vi "AdjustWaveFormsLength.vi"(4 "error in (no error)":errorcluster, 7 "AllWaveFormsIN":waveform(dbl)[](graph)) -> (0 "error out":errorcluster, 3 "AllWaveFormsOUT":waveform(dbl)[](graph))   [LabVIEW 2017]
uses:
  <vilib>/Waveform/WDTOps.llb/WDT Waveform Duration DBL.vi
  <vilib>/Waveform/WDTOps.llb/WDT Get Waveform Subset DBL.vi
  <vilib>/Waveform/WDTOps.llb/WDT Align Waveform Timestamps DBL.vi
panel:
  out "waveforms out":waveform(dbl)[](array[waveform])
  out "ShortestDuration":dbl
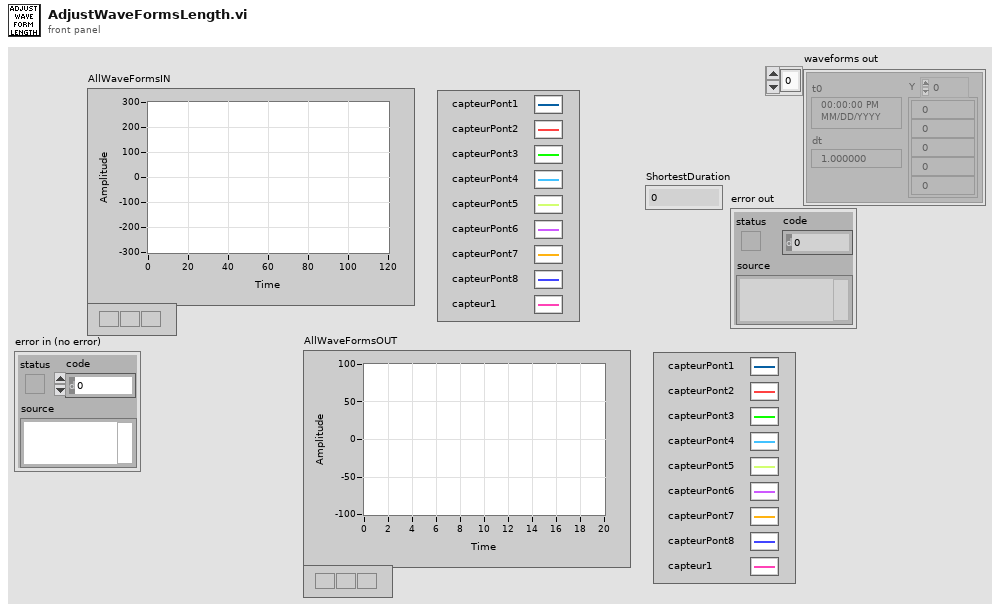
[diagram p1: front panel]
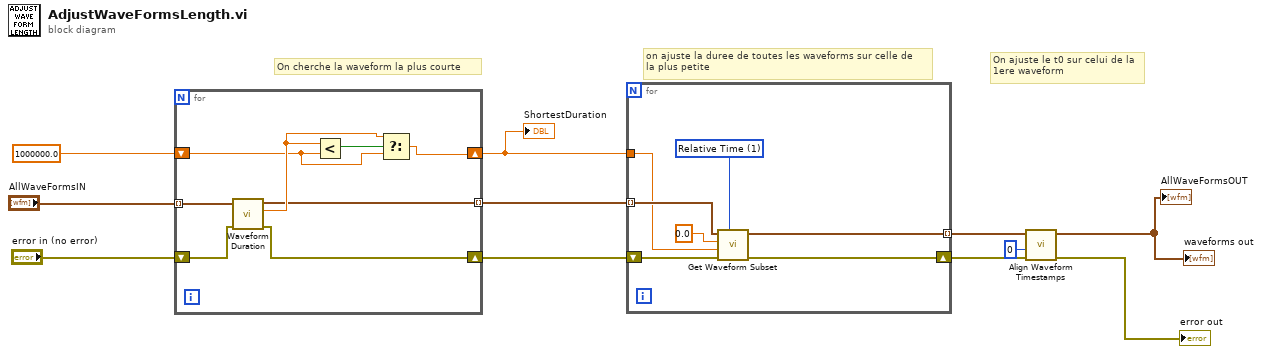
[diagram p0: block diagram]
diagram:
  # "On ajuste le t0 sur celui de la\n1ere waveform"
  # "on ajuste la duree de toutes les waveforms sur celle de\nla plus petite"
  # "On cherche la waveform la plus courte"
  n1 = for {
    tunnel: "AllWaveFormsIN" -> [w19] mode=indexing
    shift-right: [w17] -> w8
    shift-left: "error in (no error)" -> [w18]
    shift-right: [w14] -> w6
    shift-left: 1000000.0 -> [w13]
    tunnel: [w12] -> w7 mode=indexing
    n2 = call-poly <vilib>:"Waveform Duration.vi"("error in (no error)"=w18, "waveform in"=w19) -> ("error out"=w17:errorcluster, "duration"=w15:dbl, "waveform out"=w12:waveform(dbl))  [unwired: 7 in]
    n3 = Less?(x=w15, y=w13) -> (x < y?=w16:bool)
    n4 = Select(t=w15, s=w16, f=w13) -> (s? t:f=w14:dbl)
  }
  "ShortestDuration" <- w6
  n5 = for {
    shift-right: [w21] -> w5
    shift-left: w8 -> [w26]
    tunnel: w7 -> [w25] mode=indexing
    tunnel: w6 -> [w23]
    tunnel: [w20] -> w4 mode=indexing
    w22 = u16 1 items=["Samples", "Relative Time"] ("start/duration format")
    n6 = call-poly <vilib>:"Get Waveform Subset.vi"("start/duration format"=w22, "error in (no error)"=w26, "duration"=w23, "start samples/time"=0.0, "waveform in"=w25) -> ("error out"=w21:errorcluster, "waveform out"=w20:waveform(dbl))  [unwired: 1 in, 2 out]
  }
  n7 = call-poly <vilib>:"Align Waveform Timestamps.vi"("error in (no error)"=w5, "index"=0, "waveforms in"=w4) -> ("error out"=→"error out":errorcluster, "waveforms out"=→"AllWaveFormsOUT" →"waveforms out":waveform(dbl)[])  [unwired: 7 in]
